vi "Configuration Page.vi"(8 "Error in":errorcluster, 11 "INL DNL Test in":refnum<class "INL DNL Test.lvclass">=refnum) -> (0 "Error out":errorcluster, 3 "INL DNL Test out":refnum<class "INL DNL Test.lvclass">)   [LabVIEW 2020, in "INL DNL Test.lvclass"]
doc: "Configuration page to select the INL calculation method"
uses:
  INL DNL Test.lvclass
  D:/SDLC/Class/INL DNL Test/Test/Parent/Test.lvclass
  Device/Children/Children/ADC/ADC.lvclass
  Typedef/User event controls.ctl
  DNL INL Test.lvlib
panel:
  in  "Best Fit":bool caption="Best Fit method"
  in  "End Point":bool caption="End Point method"
  # "Note:\n1. Choose the method to calculate INL Result"
  # "Choose the test method"
  # "Test method"
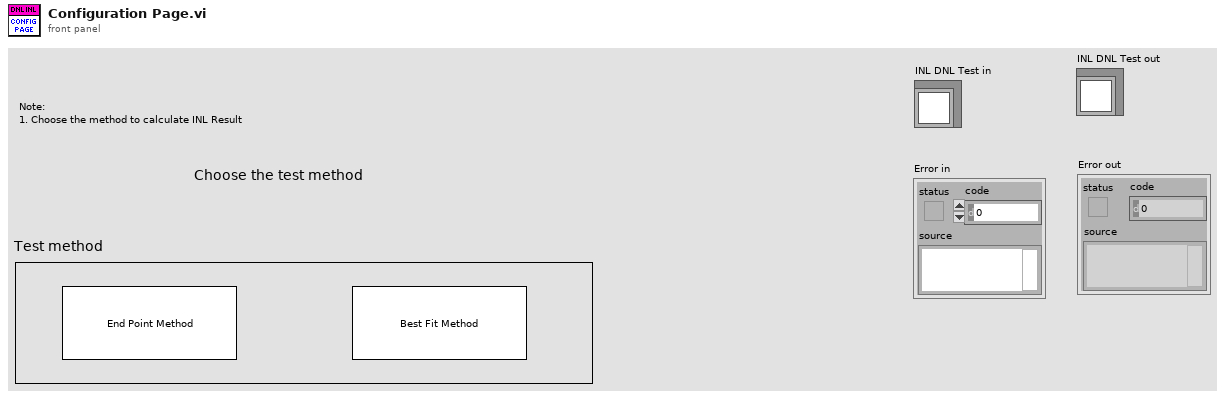
[diagram p1: front panel]
types:
  T1 = typedef "DNL INL Test.lvlib/User event controls.ctl" = enum16{"Create", "Generate", "Run Test", "Get Ref", "Destroy"}
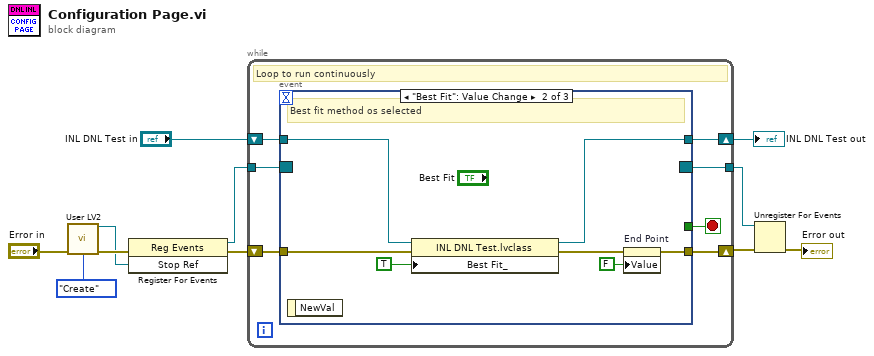
[diagram p0: block diagram]
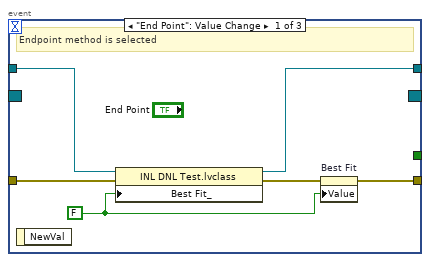
[diagram p2: hidden frame]
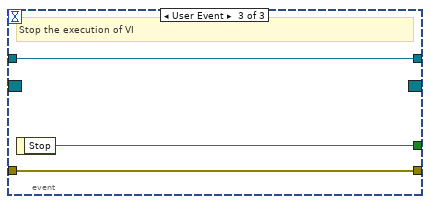
[diagram p3: hidden frame]
diagram:
  n1 = call "User LV2.vi"("Error In"="Error in", "User event controls"=User_event_controls."Create") -> ("Stop Ref"=w8:refnum<user-event>, "Error Out"=w9:errorcluster)  [unwired: 11 in, 1 out]
  n2 = register-events(error in=w9, w8) -> (reference out=w7:refnum<event-registration>, error out=w4:errorcluster)  [unwired: 1 in]
  n3 = while {
    tunnel: w7 -> [w18]
    shift-right: [w16] -> w5
    shift-left: "INL DNL Test in" -> [w17]
    shift-right: [w13] -> w2
    shift-left: w4 -> [w14]
    tunnel: [w12] -> w1
    stop <- w15 stop-if-true
    # "Loop to run continuously"
    n4 = event shown="[1] \"Best Fit\": Value Change" {
      selector: w18 -> [_ _ _]
      dyn-events: [_ _ _] -> w12
      timeout: _ -> [_ _ _]
      tunnel: [w22 w28 w32] -> w16
      tunnel: w17 -> [w23 w30 w32]
      tunnel: [_ _ w34] -> w15
      tunnel: w14 -> [w24 w31 w33]
      tunnel: [w20 w27 w33] -> w13
      event "End Point": Value Change {
        w19 = FALSE ("Best FIt_")
        # "Endpoint method is selected"
        n5 = event-data() -> ()  [unwired: 1 in, 1 out]
        n6 = property class="INL DNL Test.lvclass"(reference=w23, error in=w24, "Best Fit_"=w19) -> (reference out=w22:refnum<class "INL DNL Test.lvclass">, error out=w21:errorcluster)
        n7 = property on="Best Fit" class="Bool (strict)"(error in=w21, "Value"=w19) -> (error out=w20:errorcluster)  [unwired: 1 in, 1 out]
      }
      event "Best Fit": Value Change {
        # "Best fit method os selected"
        n8 = event-data() -> ()  [unwired: 1 in, 1 out]
        n9 = property class="INL DNL Test.lvclass"(reference=w30, error in=w31, "Best Fit_"=TRUE ("Best FIt_")) -> (reference out=w28:refnum<class "INL DNL Test.lvclass">, error out=w29:errorcluster)
        n10 = property on="End Point" class="Bool (strict)"(error in=w29, "Value"=FALSE ("End Point")) -> (error out=w27:errorcluster)  [unwired: 1 in, 1 out]
      }
      event User Event {
        # "Stop the execution of VI"
        n11 = event-data() -> ("Stop"=w34:bool)  [unwired: 1 in]
      }
    }
  }
  "INL DNL Test out" <- w5
  n12 = Unregister For Events(event registration refnum=w1, error in=w2) -> (error out=→"Error out":errorcluster)
